vi "Update Row with Results.vi"(8 "error in":errorcluster, 10 "File Info":T1, 11 "Peer Review in":refnum<class "Peer Review.lvclass">) -> (0 "error out":errorcluster, 3 "Peer Review out":refnum<class "Peer Review.lvclass">)   [LabVIEW 2020, in "Peer Review.lvclass"]
uses:
  Peer Review.lvclass
  TypeDefs/File Info.ctl
  TypeDefs/File State.ctl
  TypeDefs/VI Type.ctl
  Peer Review.lvclass/Peer Review.ctl
  <vilib>/Utility/miscctls.llb/LVRowAndColumnTypeDef.ctl
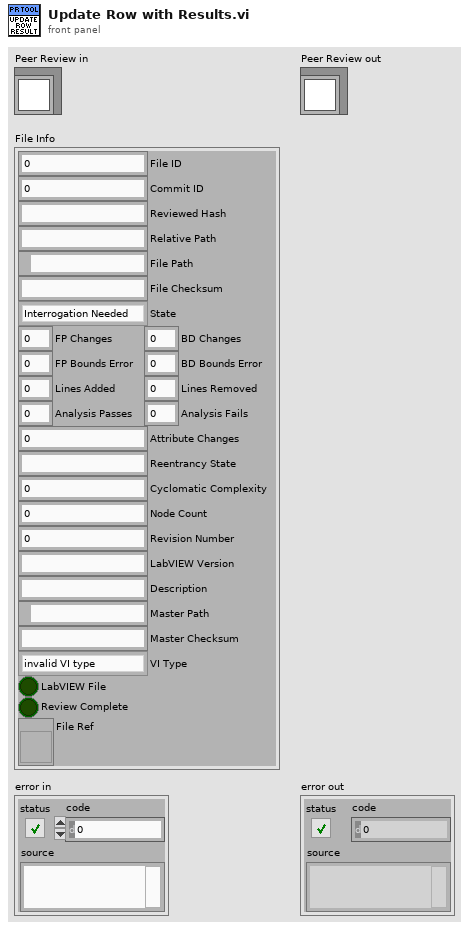
[diagram p1: front panel]
types:
  T1 = typedef "Peer Review.lvclass/File Info.ctl" = cluster{"File ID":i32, "Commit ID":i32, "Reviewed Hash":string, "Relative Path":string, "File Path":path, "File Checksum":string, "State":T2, "FP Changes":i32, "BD Changes":i32, "FP Bounds Error":dbl, "BD Bounds Error":dbl, "Lines Added":i32, "Lines Removed":i32, "Analysis Passes":i32, "Analysis Fails":i32, "Attribute Changes":i32, "Reentrancy State":string, "Cyclomatic Complexity":i32, "Node Count":i32, "Revision Number":u32, "LabVIEW Version":string, "Description":string, "Master Path":path, "Master Checksum":string, "VI Type":T3, "LabVIEW File":bool, "Review Complete":bool, "File Ref":refnum<vi>}
  T2 = typedef "Peer Review.lvclass/File State.ctl" = enum16{"Interrogation Needed", "Modified", "Deleted", "Added", "Matches Previous", "No Changes", "Moved"}
  T3 = typedef "Peer Review.lvclass/VI Type.ctl" = enum32{"invalid VI type", "Standard VI", "Control VI", "Global VI", "Polymorphic VI", "Configuration VI", "SubSystem", "Facade VI", "Method VI", "Statechart Diagram VI"}
  T4 = typedef "LVRowAndColumnTypeDef.ctl" = cluster{"Row":i32, "Column":i32}
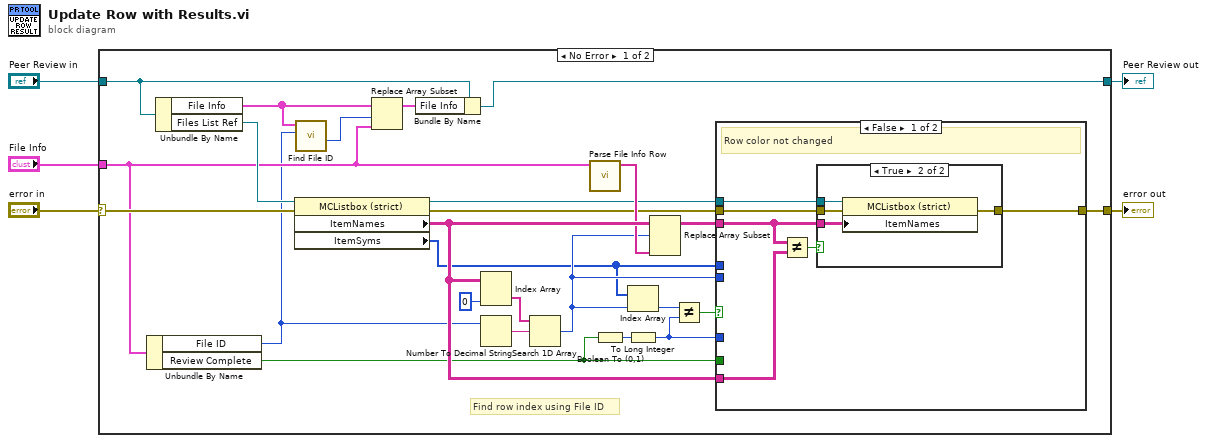
[diagram p0: block diagram]
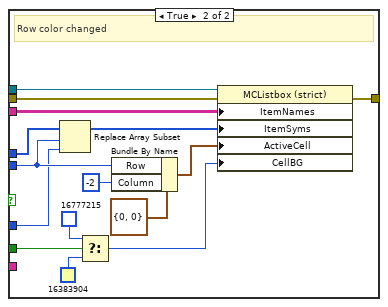
[diagram p3: hidden frame]
diagram:
  n1 = case shown="No Error" "error in" {
    selector: "error in" -> [w17 w58]
    tunnel: "File Info" -> [w13 _]
    tunnel: [w29 w58] -> w2
    tunnel: "Peer Review in" -> [w15 w57]
    tunnel: [w14 w57] -> w1
    frame No Error {
      # "Find row index using File ID"
      n2 = Unbundle By Name(w13) -> ("File ID"=w7:i32, "Review Complete"=w12:bool)
      n3 = Unbundle By Name(w15) -> ("File Info"=w9:T1[], "Files List Ref"=w28:refnum<vi>)
      n4 = property on="Property Node" class="MCListbox (strict)"(reference=w28, error in=w17) -> (reference out=w18:refnum<vi>, error out=w11:errorcluster, "ItemNames"=w21:string[][], "ItemSyms"=w6:i32[])
      n5 = call "Find File ID.vi"("File ID"=w7, "File List"=w9) -> ("Array Index"=w8:i32)  [unwired: 7 in, 2 out]
      n6 = Replace Array Subset(array=w9, new element=w13, index=w8) -> (w16:T1[])
      n7 = Bundle By Name(cluster=w15, "File Info"=w16) -> (w14:refnum<class "Peer Review.lvclass">)
      n8 = Index Array(array=w21, index (col)=0 ("disabled index (col)")) -> (element=w26:string[])  [unwired: 1 in]
      n9 = Number To Decimal String(number=w7) -> (decimal integer string=w25:string)  [unwired: 1 in]
      n10 = Search 1D Array(1D array=w26, element=w25) -> (index of element=w10:i32)  [unwired: 1 in]
      n11 = call "Parse File Info Row.vi"("File Info"=w13) -> ("Column Fields"=w19:string[])  [unwired: 10 in]
      n12 = Boolean To (0,1)(Boolean=w12) -> (0, 1=w30:i16)
      n13 = Index Array(array=w6, index=w10) -> (element=w23:i32)
      n14 = To Long Integer(number=w30) -> (32bit integer=w20:i32)
      n15 = Replace Array Subset(array=w21, new element=w19, index (row)=w10) -> (w24:string[][])  [unwired: 1 in]
      n16 = Not Equal?(x=w23, y=w20) -> (x != y?=w22:bool)
      n17 = case shown="False" w22 {
        tunnel: w11 -> [w36 w56]
        tunnel: [w34 w55] -> w29
        tunnel: w18 -> [w35 w54]
        tunnel: w24 -> [w32 w46]
        tunnel: w12 -> [_ w51]
        tunnel: w6 -> [_ w45]
        tunnel: w10 -> [_ w43]
        tunnel: w21 -> [w33 _]
        tunnel: w20 -> [_ w42]
        frame False {
          # "Row color not changed"
          n18 = Not Equal?(x=w32, y=w33) -> (x != y?=w31:bool)
          n19 = case shown="True" w31 {
            tunnel: w36 -> [w37 w41]
            tunnel: w35 -> [_ w40]
            tunnel: [w37 w39] -> w34
            tunnel: w32 -> [_ w38]
            frame False {
            }
            frame True {
              n20 = property on="Property Node" class="MCListbox (strict)"(reference=w40, error in=w41, "ItemNames"=w38) -> (error out=w39:errorcluster)  [unwired: 1 out]
            }
          }
        }
        frame True {
          # "Row color changed"
          n21 = Replace Array Subset(array=w45, new element=w42, index=w43) -> (w44:i32[])
          n22 = Select(t=u32 16777215, s=w51, f=u32 16383904) -> (s? t:f=w47:u32)
          n23 = Bundle By Name(cluster=T4 {"Row"=0, "Column"=0} ("Active Cell:Active Cell"), "Row"=w43, "Column"=-2) -> (w48:T4)
          n24 = property on="Property Node" class="MCListbox (strict)"(reference=w54, error in=w56, "ItemNames"=w46, "ItemSyms"=w44, "ActiveCell"=w48, "CellBG"=w47) -> (error out=w55:errorcluster)  [unwired: 1 out]
        }
      }
    }
    frame Error {
    }
  }
  "error out" <- w2
  "Peer Review out" <- w1
